vi "例4.17-2 实现无else的if 语句2.vi"() -> ()   [LabVIEW 2017]
panel:
  out "y":dbl
  in  "x":dbl
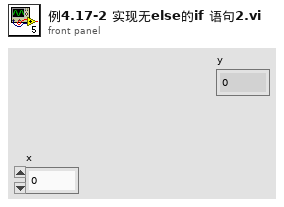
[diagram p1: front panel]
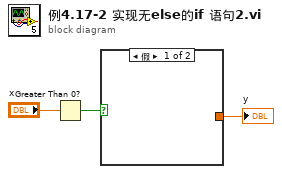
[diagram p0: block diagram]
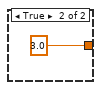
[diagram p2: hidden frame]
diagram:
  n1 = Greater Than 0?(x="x") -> (x > 0?=w3:bool)
  n2 = case shown="假" w3 {
    tunnel: [_ 3.0 ("y")] -> w1
    frame False {
    }
    frame True {
    }
  }
  "y" <- w1
